vi "instrument info parser.vi"(4 "ID":string) -> (1 "Instrument Info":string[](array[string]))   [LabVIEW 2025]
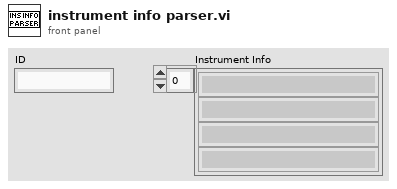
[diagram p1: front panel]
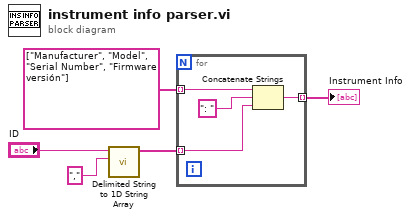
[diagram p0: block diagram]
diagram:
  n1 = call <vilib>:"Delimited String to 1D String Array.vi"("delimiter"=",", "delimited string"="ID") -> ("string array"=w3:string[])  [unwired: 9 in]
  n2 = for {
    tunnel: w3 -> [w7] mode=indexing
    tunnel: string[] ["Manufacturer", "Model", "Serial Number", "Firmware versión"] -> [w9] mode=indexing
    tunnel: [w6] -> w1 mode=indexing
    n3 = Concatenate Strings(w9, ": ", w7) -> (w6:string)
  }
  "Instrument Info" <- w1
